vi "delete channel by name.vi"(8 "error in":errorcluster, 10 "channel name":string, 11 "TDMS datalogger editor node in":refnum<class "TDMS datalogger editor node.lvclass">) -> (0 "error out":errorcluster, 3 "TDMS datalogger editor node out":refnum<class "TDMS datalogger editor node.lvclass">)   [LabVIEW 2013, in "TDMS datalogger editor node.lvclass"]
uses:
  TDMS datalogger editor node.lvclass
  <vilib>/NI/TBM Modules/TDMS Datalogger/module/configuration/TDMS datalogger configuration.lvclass
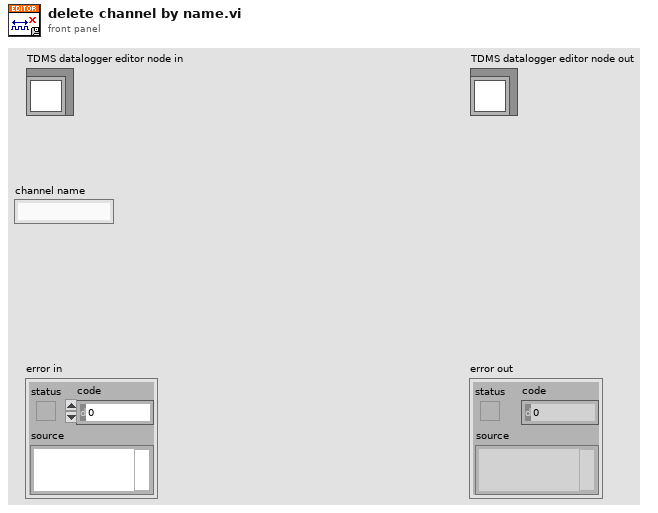
[diagram p1: front panel]
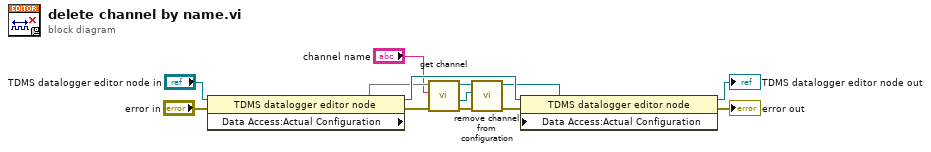
[diagram p0: block diagram]
diagram:
  n1 = property class="TDMS datalogger editor node"(reference="TDMS datalogger editor node in", error in="error in") -> (reference out=w12:refnum<class "TDMS datalogger editor node.lvclass">, error out=w5:errorcluster, "Data Access:Actual Configuration"=w10)
  n2 = call <vilib>:"get channel.vi"("error in"=w5, "name"="channel name", "module configuration in"=w10) -> ("error out"=w6:errorcluster, "channel"=w4:refnum<class "TBM channel.lvclass">, "module configuration out"=w8:refnum<class "TDMS datalogger configuration.lvclass">)  [unwired: 6 in]
  n3 = call <vilib>:"remove channel from configuration.vi"("error in"=w6, "TBM channel in"=w4, "TDMS datalogger configuration in"=w8) -> ("error out"=w3:errorcluster, "TDMS datalogger configuration out"=w7:refnum<class "TDMS datalogger configuration.lvclass">)  [unwired: 7 in]
  n4 = property class="TDMS datalogger editor node"(reference=w12, error in=w3, "Data Access:Actual Configuration"=w7) -> (reference out=→"TDMS datalogger editor node out":refnum<class "TDMS datalogger editor node.lvclass">, error out=→"error out":errorcluster)
